vi "Teleop Intake Control.vi"(9 "D-Pad":T2, 10 "Button Cluster":T3, 11 "Axes":T1) -> ()   [LabVIEW 2016]
uses:
  Common Code/Gamepads/Button Cluster.ctl
  Common Code/Gamepads/D-Pad.ctl
  Common Code/Gamepads/Axes Cluster.ctl
  Robot Global Data.vi
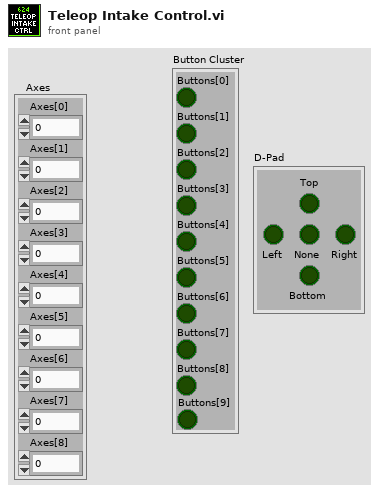
[diagram p1: front panel]
types:
  T1 = typedef "Axes Cluster.ctl" = cluster{"Axes[0]":dbl, "Axes[1]":dbl, "Axes[2]":dbl, "Axes[3]":dbl, "Axes[4]":dbl, "Axes[5]":dbl, "Axes[6]":dbl, "Axes[7]":dbl, "Axes[8]":dbl}
  T2 = typedef "D-Pad.ctl" = cluster{"Top":bool, "Bottom":bool, "None":bool, "Right":bool, "Left":bool}
  T3 = typedef "Button Cluster.ctl" = cluster{"Buttons[0]":bool, "Buttons[1]":bool, "Buttons[2]":bool, "Buttons[3]":bool, "Buttons[4]":bool, "Buttons[5]":bool, "Buttons[6]":bool, "Buttons[7]":bool, "Buttons[8]":bool, "Buttons[9]":bool}
  T4 = typedef "Dashboard Control Data.ctl" = cluster{"Drivetrain Settings":T5, "Intake Presets ":T7, "Drivetrain Encoder Settings":T8, "Shooter Settings":T9, "Intake Settings":T10}
  T5 = typedef "Drivetrain Settings.ctl" = cluster{"Gyro Tolerance":dbl, "Gyro Steer PID Gains":T6, "Y Power Multiplier":dbl, "Turn Power Multiplier":dbl, "Gyro Output":dbl, "Creep Rate":dbl, "Distance Drive PID Gains":T6, "Distance Tolerance":dbl, "Distance Output":dbl, "Strafe Threshold":dbl, "Strafe Correct":bool, "Strafe Corect Tolerance":dbl, "Translate Drive PID Gains":T6, "Strafe Output":dbl}
  T6 = typedef "PID Gains.ctl" = cluster{"proportional gain (Kc)":dbl, "integral time (Ti, min)":dbl, "derivative time (Td, min)":dbl}
  T7 = typedef "Intake Presets.ctl" = cluster{"Intake Speed ":dbl, "Outake Speed":dbl, "Set Time":dbl}
  T8 = typedef "Drivetrain Encoder Settings.ctl" = cluster{"Left Tick Constant":dbl, "Right Tick Contant":dbl, "Reset Encoders":bool, "Center Tick Constant":dbl}
  T9 = typedef "Shooter Settings.ctl" = cluster{"Key Output":dbl, "Airship Output":dbl, "Trigger Power":dbl}
  T10 = typedef "Intake Settings.ctl" = cluster{"Motor Output":dbl}
  T11 = typedef "Intake Control Cluster.ctl" = cluster{"Intake Modes":T12, "Override IR":bool, "Intake Auto States":T13, "Intake Motor  Output":dbl}
  T12 = typedef "Intake Modes.ctl" = enum16{"Manual", "Auto"}
  T13 = typedef "Intake Auto States.ctl" = enum16{"Idle", "Load Ball", "Load Gear", "Outake Gear", "Outake Ball"}
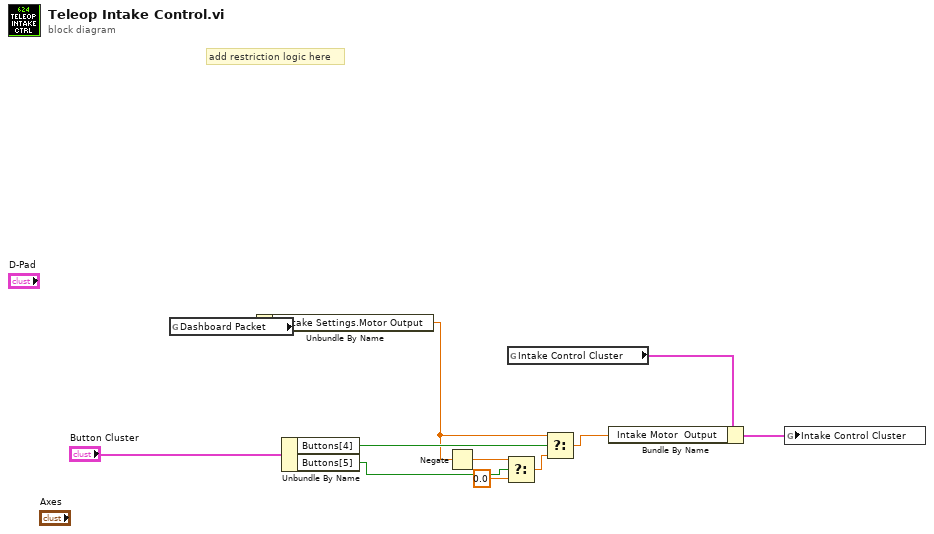
[diagram p0: block diagram]
diagram:
  # "add restriction logic here"
  n1 = global read "Robot Global Data.vi" "Dashboard Packet"() -> (w3:T4)
  n2 = Unbundle By Name(w3) -> ("Intake Settings.Motor Output"=w2:dbl)
  n3 = Unbundle By Name("Button Cluster") -> ("Buttons[4]"=w10:bool, "Buttons[5]"=w8:bool)
  n4 = Negate(x=w2) -> (-x=w1:dbl)
  n5 = Select(t=w1, s=w8, f=0.0) -> (s? t:f=w9:dbl)
  n6 = global read "Robot Global Data.vi" "Intake Control Cluster"() -> (w7:T11)
  n7 = Select(t=w2, s=w10, f=w9) -> (s? t:f=w6:dbl)
  n8 = Bundle By Name(cluster=w7, "Intake Motor  Output"=w6) -> (w5:T11)
  n9 = global write "Robot Global Data.vi" "Intake Control Cluster"(w5) -> ()
